vi "Configure Measurement Cursors.vi"(11 "State in":T2={"Graph Visible Items"={"Plot Legend"=FALSE, "Scale Legend"=FALSE, "Graph Palette"=FALSE, "Cursor Legend"=FALSE, "X Scrollbar"=FALSE}, "View Table"=FALSE, "Table Visible Items"={"Vertical Scrollbar"=FALSE, "Horizontal Scrollbar"=FALSE, "Row Headers"=FALSE, "Column Headers"=FALSE, "Vertical Lines"=FALSE, "Horizontal Lines"=FALSE}, "Header Font"={"Font Name"="", "Size"=0, "Bold"=FALSE, "Italic"=FALSE, "Underline"=FALSE, "Strikeout"=FALSE, "Color"=0}, "Cell Font"={"Font Name"="", "Size"=0, "Bold"=FALSE, "Italic"=FALSE, "Underline"=FALSE, "Strikeout"=FALSE, "Color"=0}, "Description and Tip..."={"Description"="", "Tip"=""}, "Moveable Splitter Position"=0, "Measurement Cursor Configuration"={"XY"={"enable XY"=FALSE, "Position (X)"=[], "Type"=enum."Absolute", "Y reference"=0.0, "color"=0}, "band"={"enable band"=FALSE, "B1"=0.0, "B2"=0.0, "Fixed bandwidth (B2-B1)"=0.0, "B1 color"=0, "B2 color"=0}, "harmonic"={"enable harmonics"=FALSE, "X reference (1X)"=0.0, "Maximum"=0, "Subset"=enum."All", "1X color"=0, "MX color"=0}, "sideband"={"enable sideband"=FALSE, "X center (C)"=0.0, "Sidebands"=0, "X spacing (s)"=0.0, "Center color"=0, "Sideband color"=0}}, "Cursors"={"List"=[], "Tags"=[]}, "X Increment"=0.0, "X Scale"={"Label Visible"=FALSE, "Label Text"="", "Mapping Mode"=0, "Format String"=""}, "Y Scale"={"Label Visible"=FALSE, "Label Text"="", "Mapping Mode"=0, "Format String"=""}, "Colors"={"background"=16777215, "major grid"=8355711, "minor grid"=12632256, "font"=0}, "desired spectrum view"={"scaling"={"linear/dB"=enum."no change", "dB reference"=0.0, "power/magnitude"=enum."no change", "view"=enum."no change"}, "spectral density"=enum."no change"}, "Plot Color Wheel"=[3381759, 32768, 982784, 4375295, 13827953, 13457919, 16757522, 4343295, 16728758, 12095254], "Plots"=[], "registered user events"=variant, "Lock 1X to Peak"=FALSE} caption="State" {"Y Scale"."Mapping Mode" items=["Linear", "Logarithmic", "dB"]; "X Scale"."Mapping Mode" items=["Linear", "Logarithmic"]}) -> (1 "OK":bool, 3 "State out":T2={"Graph Visible Items"={"Plot Legend"=FALSE, "Scale Legend"=FALSE, "Graph Palette"=FALSE, "Cursor Legend"=FALSE, "X Scrollbar"=FALSE}, "View Table"=FALSE, "Table Visible Items"={"Vertical Scrollbar"=FALSE, "Horizontal Scrollbar"=FALSE, "Row Headers"=FALSE, "Column Headers"=FALSE, "Vertical Lines"=FALSE, "Horizontal Lines"=FALSE}, "Header Font"={"Font Name"="", "Size"=0, "Bold"=FALSE, "Italic"=FALSE, "Underline"=FALSE, "Strikeout"=FALSE, "Color"=0}, "Cell Font"={"Font Name"="", "Size"=0, "Bold"=FALSE, "Italic"=FALSE, "Underline"=FALSE, "Strikeout"=FALSE, "Color"=0}, "Description and Tip..."={"Description"="", "Tip"=""}, "Moveable Splitter Position"=0, "Measurement Cursor Configuration"={"XY"={"enable XY"=FALSE, "Position (X)"=[], "Type"=enum."Absolute", "Y reference"=0.0, "color"=0}, "band"={"enable band"=FALSE, "B1"=0.0, "B2"=0.0, "Fixed bandwidth (B2-B1)"=0.0, "B1 color"=0, "B2 color"=0}, "harmonic"={"enable harmonics"=FALSE, "X reference (1X)"=0.0, "Maximum"=0, "Subset"=enum."All", "1X color"=0, "MX color"=0}, "sideband"={"enable sideband"=FALSE, "X center (C)"=0.0, "Sidebands"=0, "X spacing (s)"=0.0, "Center color"=0, "Sideband color"=0}}, "Cursors"={"List"=[], "Tags"=[]}, "X Increment"=0.0, "X Scale"={"Label Visible"=FALSE, "Label Text"="", "Mapping Mode"=0, "Format String"=""}, "Y Scale"={"Label Visible"=FALSE, "Label Text"="", "Mapping Mode"=0, "Format String"=""}, "Colors"={"background"=16777215, "major grid"=8355711, "minor grid"=12632256, "font"=0}, "desired spectrum view"={"scaling"={"linear/dB"=enum."no change", "dB reference"=0.0, "power/magnitude"=enum."no change", "view"=enum."no change"}, "spectral density"=enum."no change"}, "Plot Color Wheel"=[3381759, 32768, 982784, 4375295, 13827953, 13457919, 16757522, 4343295, 16728758, 12095254], "Plots"=[], "registered user events"=variant, "Lock 1X to Peak"=FALSE} caption="State" {"Y Scale"."Mapping Mode" items=["Linear", "Logarithmic", "dB"]; "X Scale"."Mapping Mode" items=["Linear", "Logarithmic"]})   [LabVIEW 2017, in "Octave with Cursors.xctl"]
doc: "Dialog for cursor configuration."
uses:
  <vilib>/addons/_XControls/Octave with Cursors/Octave with Cursors.xctl
  <vilib>/addons/_XControls/Octave with Cursors/Controls/State.ctl
  <vilib>/Utility/miscctls.llb/LVFontTypeDef.ctl
  <vilib>/addons/_XControls/Octave with Cursors/Controls/Measurement Cursor Configuration.ctl
panel:
  in  "XY color":u32(colorbox)
  in  "enable XY":bool
  in  "Type":enum16{"Absolute", "Relative"}(ring)
  in  "Position (i)":dbl[](array[numeric]) min=0.0 step=1.0
  in  "Y reference":dbl
  in  "B2 color":u32(colorbox)
  in  "B1 color":u32(colorbox)
  in  "Fixed ratio (octaves)":T1(ring)
  in  "enable band":bool
  in  "Stop (b2)":dbl=480.0
  in  "Start (b1)":dbl=20.0
  in  "1X color":u32(colorbox)
  in  "MX color":u32(colorbox)
  in  "enable harmonics":bool
  in  "Maximum (mX)":i32=10 min=2 max=99 step=1
  in  "X reference (1X)":dbl=60.0 min=0.001 step=1.0
  in  "Subset":enum16{"All", "Even", "Odd"}(ring)
  in  "Center color":u32(colorbox)
  in  "Sideband color":u32(colorbox)
  in  "Sidebands (sn)":i32=2 min=1 max=9 step=1
  in  "enable sideband":bool
  in  "X spacing (s)":dbl=60.0 min=0.0 step=1.0
  in  "X center (C)":dbl=8000.0 min=0.001 step=0.001
  in  "Cancel":bool
  in  "OK":bool
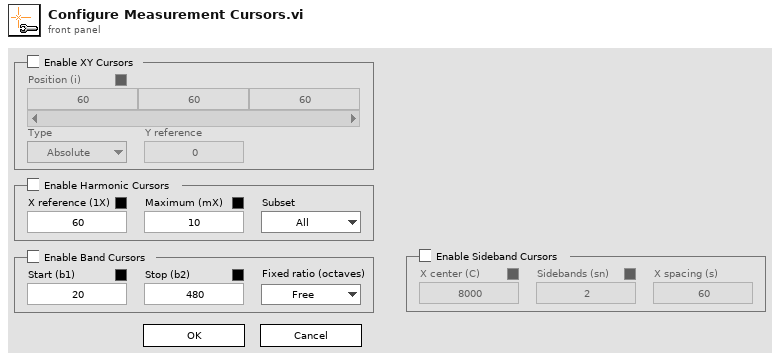
[diagram p1: front panel]
types:
  T1 = enum16{"Free", "1/24", "1/12", "1/6", "1/3", "1", "2", "4", "6", "8", "10"}
  T2 = typedef "Octave with Cursors.xctl/State.ctl" = cluster{"Graph Visible Items":cluster{"Plot Legend":bool, "Scale Legend":bool, "Graph Palette":bool, "Cursor Legend":bool, "X Scrollbar":bool}, "View Table":bool, "Table Visible Items":cluster{"Vertical Scrollbar":bool, "Horizontal Scrollbar":bool, "Row Headers":bool, "Column Headers":bool, "Vertical Lines":bool, "Horizontal Lines":bool}, "Header Font":T3, "Cell Font":T3, "Description and Tip...":cluster{"Description":string, "Tip":string}, "Moveable Splitter Position":i32, "Measurement Cursor Configuration":T4, "Cursors":cluster{"List":cluster{"Name":string, "Color":u32, "Style":i32, "Point Style":u8, "Name Visible":bool, "Allow Drag":bool, "Cursor Mode":u32, "Plot":i32, "Index":i32, "Position":cluster{"X":dbl, "Y":dbl}, "X Scale":u32, "Y Scale":u32, "Watch Plots":i32[], "Watch All Plots":bool, "Plot Area":i32, "Label Offset":cluster{"X":dbl, "Y":dbl}}[], "Tags":variant[]}, "X Increment":dbl, "X Scale":cluster{"Label Visible":bool, "Label Text":string, "Mapping Mode":u8, "Format String":string}, "Y Scale":cluster{"Label Visible":bool, "Label Text":string, "Mapping Mode":u8, "Format String":string}, "Colors":cluster{"background":u32, "major grid":u32, "minor grid":u32, "font":u32}, "desired spectrum view":cluster{"scaling":cluster{"linear/dB":enum16{"no change", "linear", "dB"}, "dB reference":dbl, "power/magnitude":enum16{"no change", "power", "magnitude"}, "view":enum16{"no change", "rms", "peak", "peak-peak"}}, "spectral density":enum16{"no change", "spectrum", "spectral density"}}, "Plot Color Wheel":u32[], "Plots":cluster{"Name":string, "Line Color":u32, "Line Style":u8, "Line Width":u8, "Fill/Point Color":u32, "Point Style":u8, "Fill To":i16, "Interpolation":u8, "Anti-aliased":bool}[], "registered user events":variant, "Lock 1X to Peak":bool}
  T3 = typedef "LVFontTypeDef.ctl" = cluster{"Font Name":string, "Size":u16, "Bold":bool, "Italic":bool, "Underline":bool, "Strikeout":bool, "Color":u32}
  T4 = typedef "Octave with Cursors.xctl/Measurement Cursor Configuration.ctl" = cluster{"XY":cluster{"enable XY":bool, "Position (X)":dbl[], "Type":enum16{"Absolute", "Relative"}, "Y reference":dbl, "color":u32}, "band":cluster{"enable band":bool, "B1":dbl, "B2":dbl, "Fixed bandwidth (B2-B1)":dbl, "B1 color":u32, "B2 color":u32}, "harmonic":cluster{"enable harmonics":bool, "X reference (1X)":dbl, "Maximum":i32, "Subset":enum16{"All", "Even", "Odd"}, "1X color":u32, "MX color":u32}, "sideband":cluster{"enable sideband":bool, "X center (C)":dbl, "Sidebands":i32, "X spacing (s)":dbl, "Center color":u32, "Sideband color":u32}}
  T5 = cluster{"enable XY":bool, "Position (X)":dbl[], "Type":enum16{"Absolute", "Relative"}, "Y reference":dbl, "color":u32}
  T6 = cluster{"enable harmonics":bool, "X reference (1X)":dbl, "Maximum":i32, "Subset":enum16{"All", "Even", "Odd"}, "1X color":u32, "MX color":u32}
  T7 = cluster{"enable sideband":bool, "X center (C)":dbl, "Sidebands":i32, "X spacing (s)":dbl, "Center color":u32, "Sideband color":u32}
  T8 = cluster{"enable band":bool, "B1":dbl, "B2":dbl, "Fixed bandwidth (B2-B1)":dbl, "B1 color":u32, "B2 color":u32}
  T9 = enum8{"Enabled", "Disabled", "Disabled and Grayed Out"}
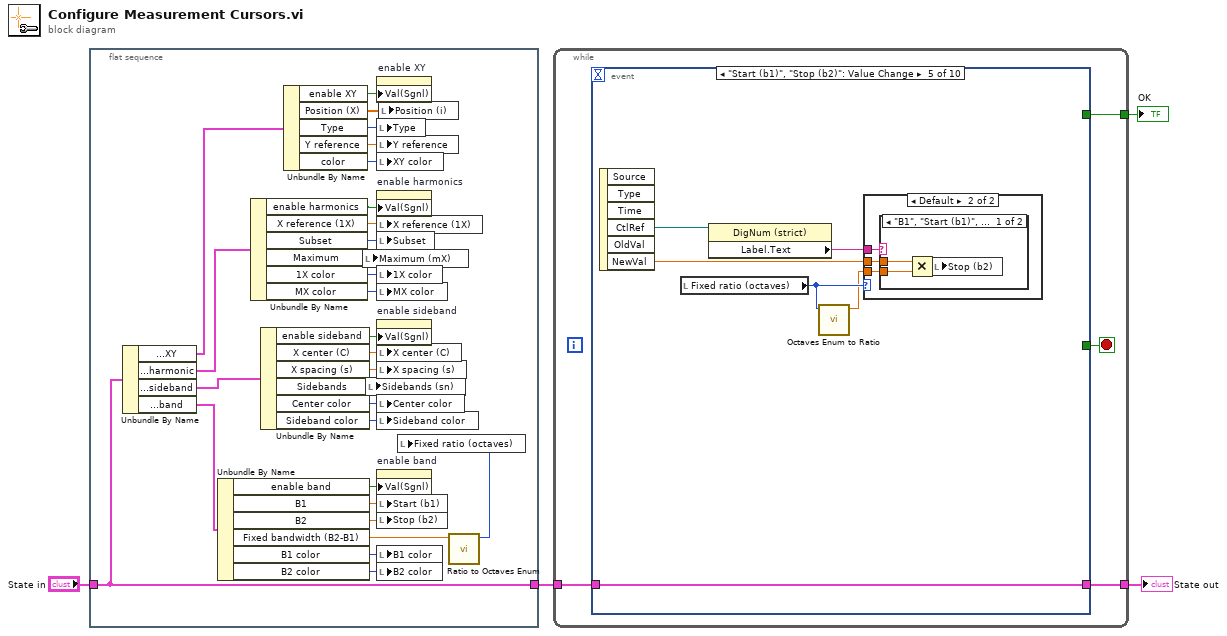
[diagram p0: block diagram]
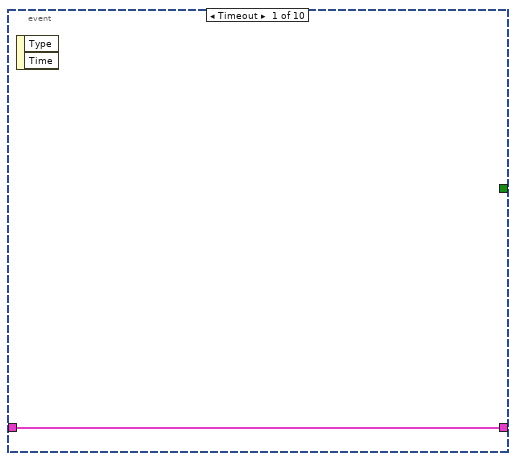
[diagram p2: hidden frame]
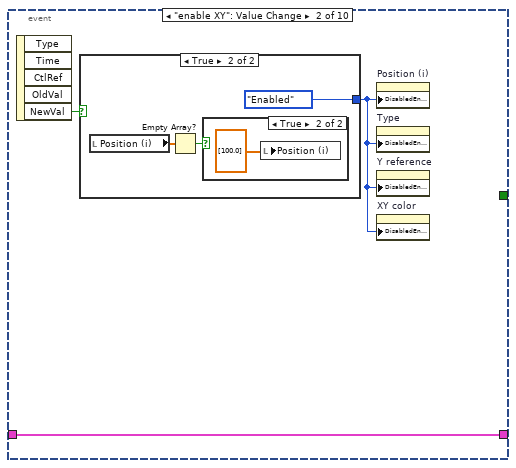
[diagram p3: hidden frame]
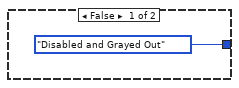
[diagram p4: hidden frame]
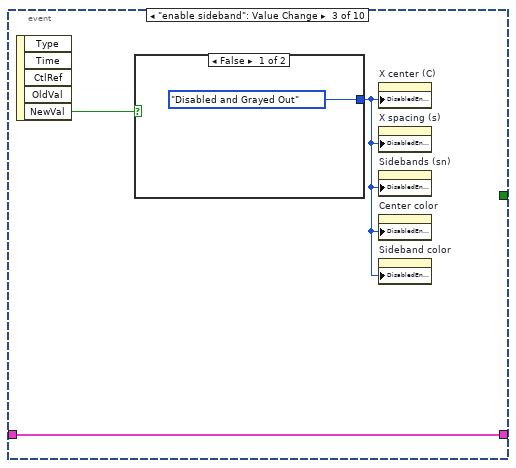
[diagram p6: hidden frame]
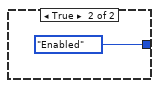
[diagram p7: hidden frame]
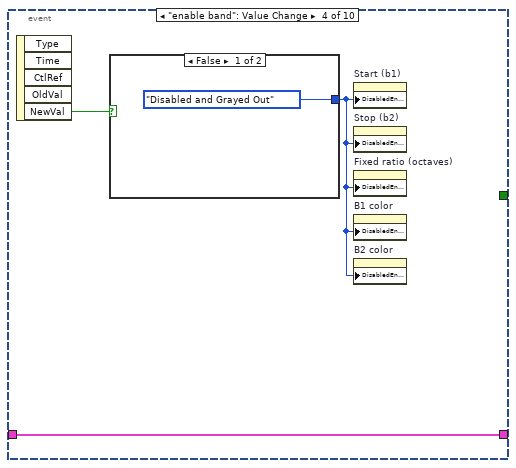
[diagram p8: hidden frame]
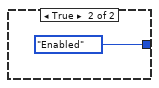
[diagram p9: hidden frame]
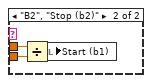
[diagram p11: hidden frame]
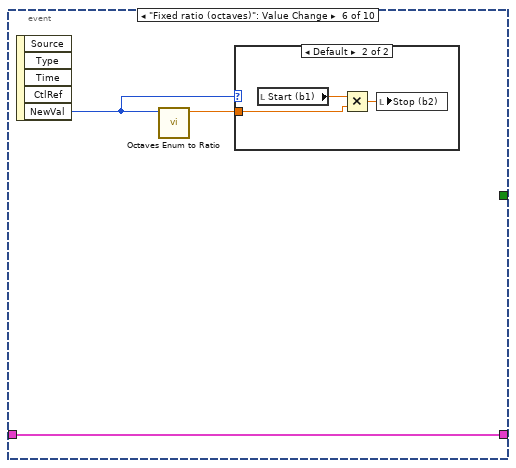
[diagram p12: hidden frame]
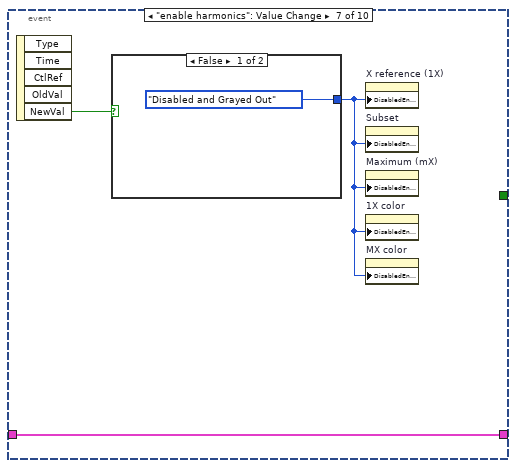
[diagram p14: hidden frame]
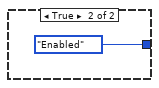
[diagram p15: hidden frame]
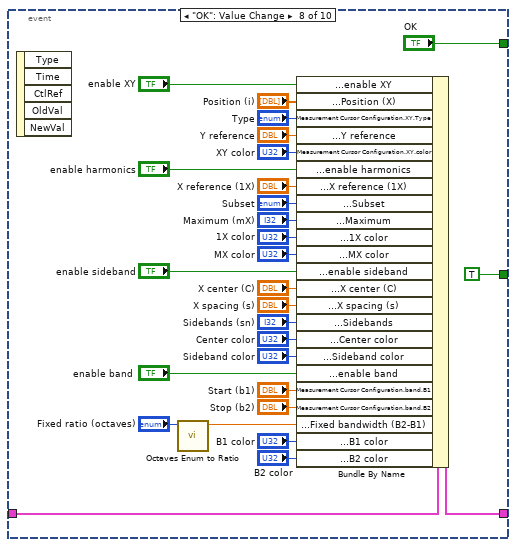
[diagram p16: hidden frame]
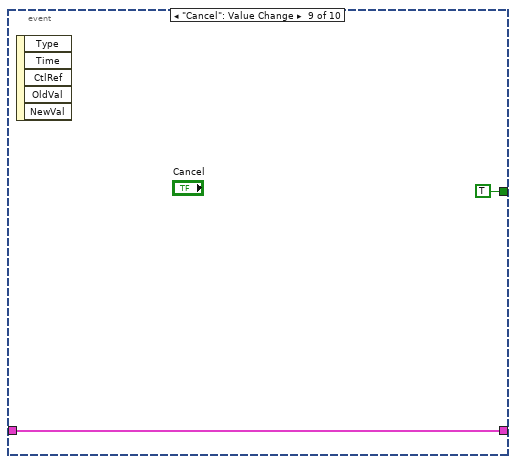
[diagram p17: hidden frame]
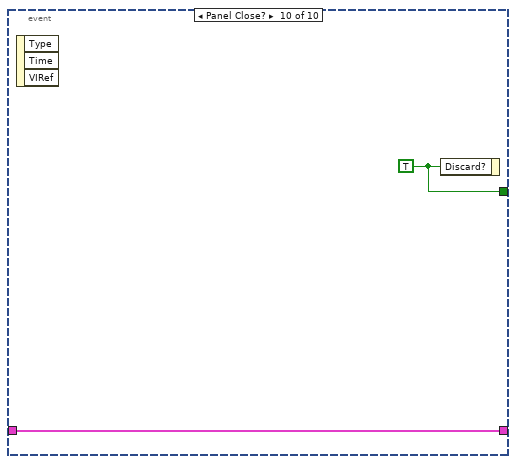
[diagram p18: hidden frame]
diagram:
  n1 = flat-sequence {
    tunnel: "State in" -> [w18]
    tunnel: [w18] -> w2
    frame #0 {
      n2 = Unbundle By Name(w18) -> ("Measurement Cursor Configuration.XY"=w33:T5, "Measurement Cursor Configuration.harmonic"=w29:T6, "Measurement Cursor Configuration.sideband"=w25:T7, "Measurement Cursor Configuration.band"=w21:T8)
      n3 = Unbundle By Name(w21) -> ("enable band"=w14:bool, "B1"=w20:dbl, "B2"=w19:dbl, "Fixed bandwidth (B2-B1)"=w6:dbl, "B1 color"=w8:u32, "B2 color"=w7:u32)
      n4 = Unbundle By Name(w29) -> ("enable harmonics"=w16:bool, "X reference (1X)"=w28:dbl, "Subset"=w27:enum16{"All", "Even", "Odd"}, "Maximum"=w26:i32, "1X color"=w12:u32, "MX color"=w11:u32)
      n5 = Unbundle By Name(w25) -> ("enable sideband"=w15:bool, "X center (C)"=w24:dbl, "X spacing (s)"=w23:dbl, "Sidebands"=w22:i32, "Center color"=w10:u32, "Sideband color"=w9:u32)
      n6 = Unbundle By Name(w33) -> ("enable XY"=w17:bool, "Position (X)"=w32:dbl[], "Type"=w31:enum16{"Absolute", "Relative"}, "Y reference"=w30:dbl, "color"=w13:u32)
      n7 = local write "Maximum (mX)"(w26) -> ()
      n8 = local write "Sidebands (sn)"(w22) -> ()
      n9 = property on="enable XY" class="Bool (strict)"("Val(Sgnl)"=w17) -> ()  [unwired: 2 in, 2 out]
      n10 = local write "Type"(w31) -> ()
      n11 = local write "Y reference"(w30) -> ()
      n12 = local write "XY color"(w13) -> ()
      n13 = property on="enable harmonics" class="Bool (strict)"("Val(Sgnl)"=w16) -> ()  [unwired: 2 in, 2 out]
      n14 = local write "X reference (1X)"(w28) -> ()
      n15 = local write "Subset"(w27) -> ()
      n16 = local write "1X color"(w12) -> ()
      n17 = local write "MX color"(w11) -> ()
      n18 = property on="enable sideband" class="Bool (strict)"("Val(Sgnl)"=w15) -> ()  [unwired: 2 in, 2 out]
      n19 = local write "X center (C)"(w24) -> ()
      n20 = local write "X spacing (s)"(w23) -> ()
      n21 = local write "Center color"(w10) -> ()
      n22 = local write "Sideband color"(w9) -> ()
      n23 = property on="enable band" class="Bool (strict)"("Val(Sgnl)"=w14) -> ()  [unwired: 2 in, 2 out]
      n24 = local write "Start (b1)"(w20) -> ()
      n25 = local write "Stop (b2)"(w19) -> ()
      n26 = local write "B1 color"(w8) -> ()
      n27 = local write "B2 color"(w7) -> ()
      n28 = local write "Position (i)"(w32) -> ()
      n29 = call <vilib>:"Ratio to Octaves Enum.vi"("ratio"=w6) -> ("octaves"=w5:T1)  [unwired: 10 in]
      n30 = local write "Fixed ratio (octaves)"(w5) -> ()
    }
  }
  n31 = while {
    tunnel: w2 -> [w35]
    tunnel: [w36] -> w4
    tunnel: [w34] -> w1
    stop <- w37 stop-if-true
    n32 = event shown="[4] \"Start (b1)\", \"Stop (b2)\": Value Change" {
      selector: _ -> [_ _ _ _ _ _ _ _ _ _]
      dyn-events: _ -> [_ _ _ _ _ _ _ _ _ _]
      timeout: _ -> [_ _ _ _ _ _ _ _ _ _]
      tunnel: [_ _ _ _ _ _ _ TRUE TRUE w113] -> w37
      tunnel: [w38 w40 w48 w53 w62 w74 w79 w96 w111 w114] -> w36
      tunnel: w35 -> [w38 w40 w48 w53 w62 w74 w79 w97 w111 w114]
      tunnel: [_ _ _ _ _ _ _ "OK" _ _] -> w34
      event Timeout {
        n33 = event-data() -> ()  [unwired: 1 in, 2 out]
      }
      event "enable XY": Value Change {
        n34 = event-data() -> ("NewVal"=w41:bool)  [unwired: 1 in, 4 out]
        n35 = case shown="True" w41 {
          tunnel: [T9."Disabled and Grayed Out" ("Disabled") T9."Enabled" ("Disabled")] -> w39
          frame False {
          }
          frame True {
            n36 = local read "Position (i)"() -> (w44:dbl[])
            n37 = Empty Array?(array=w44) -> (empty?=w43:bool)
            n38 = case shown="True" w43 {
              frame False {
              }
              frame True {
                n39 = local write "Position (i)"(dbl[] [100.0] ("Position (i)")) -> ()
              }
            }
          }
        }
        n40 = property on="Position (i)" class="Arr (strict)"("DisabledEnum"=w39) -> ()  [unwired: 2 in, 2 out]
        n41 = property on="Type" class="Enum (strict)"("DisabledEnum"=w39) -> ()  [unwired: 2 in, 2 out]
        n42 = property on="Y reference" class="DigNum (strict)"("DisabledEnum"=w39) -> ()  [unwired: 2 in, 2 out]
        n43 = property on="XY color" class="ColBox"("DisabledEnum"=w39) -> ()  [unwired: 2 in, 2 out]
      }
      event "enable sideband": Value Change {
        n44 = event-data() -> ("NewVal"=w49:bool)  [unwired: 1 in, 4 out]
        n45 = case shown="False" w49 {
          tunnel: [T9."Disabled and Grayed Out" ("Disabled") T9."Enabled" ("Disabled")] -> w47
          frame False {
          }
          frame True {
          }
        }
        n46 = property on="X center (C)" class="DigNum (strict)"("DisabledEnum"=w47) -> ()  [unwired: 2 in, 2 out]
        n47 = property on="X spacing (s)" class="DigNum (strict)"("DisabledEnum"=w47) -> ()  [unwired: 2 in, 2 out]
        n48 = property on="Sidebands (sn)" class="DigNum (strict)"("DisabledEnum"=w47) -> ()  [unwired: 2 in, 2 out]
        n49 = property on="Center color" class="ColBox"("DisabledEnum"=w47) -> ()  [unwired: 2 in, 2 out]
        n50 = property on="Sideband color" class="ColBox"("DisabledEnum"=w47) -> ()  [unwired: 2 in, 2 out]
      }
      event "enable band": Value Change {
        n51 = event-data() -> ("NewVal"=w54:bool)  [unwired: 1 in, 4 out]
        n52 = case shown="False" w54 {
          tunnel: [T9."Disabled and Grayed Out" ("Disabled") T9."Enabled" ("Disabled")] -> w52
          frame False {
          }
          frame True {
          }
        }
        n53 = property on="Start (b1)" class="DigNum (strict)"("DisabledEnum"=w52) -> ()  [unwired: 2 in, 2 out]
        n54 = property on="Stop (b2)" class="DigNum (strict)"("DisabledEnum"=w52) -> ()  [unwired: 2 in, 2 out]
        n55 = property on="Fixed ratio (octaves)" class="Enum (strict)"("DisabledEnum"=w52) -> ()  [unwired: 2 in, 2 out]
        n56 = property on="B1 color" class="ColBox"("DisabledEnum"=w52) -> ()  [unwired: 2 in, 2 out]
        n57 = property on="B2 color" class="ColBox"("DisabledEnum"=w52) -> ()  [unwired: 2 in, 2 out]
      }
      event "Start (b1)", "Stop (b2)": Value Change {
        n58 = event-data() -> ("CtlRef"=w60:refnum<vi>, "NewVal"=w59:dbl)  [unwired: 1 in, 4 out]
        n59 = local read "Fixed ratio (octaves)"() -> (w58:T1)
        n60 = property class="DigNum (strict)"(reference=w60) -> ("Label.Text"=w61:string)  [unwired: 1 in, 2 out]
        n61 = call <vilib>:"Octaves Enum to Ratio.vi"("octaves"=w58) -> ("ratio"=w57:dbl)  [unwired: 10 in]
        n62 = case shown="Default" w58 {
          tunnel: w61 -> [_ w65]
          tunnel: w59 -> [_ w64]
          tunnel: w57 -> [_ w63]
          frame "Free" {
          }
          frame Default {
            n63 = case shown="\"B1\", \"Start (b1)\", Default" w65 {
              tunnel: w64 -> [w68 w71]
              tunnel: w63 -> [w67 w70]
              frame "B1", "Start (b1)", Default {
                n64 = Multiply(x=w68, y=w67) -> (x*y=w66:dbl)
                n65 = local write "Stop (b2)"(w66) -> ()
              }
              frame "B2", "Stop (b2)" {
                n66 = Divide(x=w71, y=w70) -> (x/y=w69:dbl)
                n67 = local write "Start (b1)"(w69) -> ()
              }
            }
          }
        }
      }
      event "Fixed ratio (octaves)": Value Change {
        n68 = event-data() -> ("NewVal"=w72:T1)  [unwired: 1 in, 4 out]
        n69 = call <vilib>:"Octaves Enum to Ratio.vi"("octaves"=w72) -> ("ratio"=w73:dbl)  [unwired: 10 in]
        n70 = case shown="Default" w72 {
          tunnel: w73 -> [_ w77]
          frame "Free" {
          }
          frame Default {
            n71 = local read "Start (b1)"() -> (w76:dbl)
            n72 = Multiply(x=w76, y=w77) -> (x*y=w75:dbl)
            n73 = local write "Stop (b2)"(w75) -> ()
          }
        }
      }
      event "enable harmonics": Value Change {
        n74 = event-data() -> ("NewVal"=w80:bool)  [unwired: 1 in, 4 out]
        n75 = case shown="False" w80 {
          tunnel: [T9."Disabled and Grayed Out" ("Disabled") T9."Enabled" ("Disabled")] -> w78
          frame False {
          }
          frame True {
          }
        }
        n76 = property on="X reference (1X)" class="DigNum (strict)"("DisabledEnum"=w78) -> ()  [unwired: 2 in, 2 out]
        n77 = property on="Subset" class="Enum (strict)"("DisabledEnum"=w78) -> ()  [unwired: 2 in, 2 out]
        n78 = property on="Maximum (mX)" class="DigNum (strict)"("DisabledEnum"=w78) -> ()  [unwired: 2 in, 2 out]
        n79 = property on="1X color" class="ColBox"("DisabledEnum"=w78) -> ()  [unwired: 2 in, 2 out]
        n80 = property on="MX color" class="ColBox"("DisabledEnum"=w78) -> ()  [unwired: 2 in, 2 out]
      }
      event "OK": Value Change {
        n81 = event-data() -> ()  [unwired: 1 in, 5 out]
        n82 = call <vilib>:"Octaves Enum to Ratio.vi"("octaves"="Fixed ratio (octaves)") -> ("ratio"=w83:dbl)  [unwired: 10 in]
        n83 = Bundle By Name(cluster=w97, "Measurement Cursor Configuration.XY.enable XY"="enable XY", "Measurement Cursor Configuration.XY.Position (X)"="Position (i)", "Measurement Cursor Configuration.XY.Type"="Type", "Measurement Cursor Configuration.XY.Y reference"="Y reference", "Measurement Cursor Configuration.XY.color"="XY color", "Measurement Cursor Configuration.harmonic.enable harmonics"="enable harmonics", "Measurement Cursor Configuration.harmonic.X reference (1X)"="X reference (1X)", "Measurement Cursor Configuration.harmonic.Subset"="Subset", "Measurement Cursor Configuration.harmonic.Maximum"="Maximum (mX)", "Measurement Cursor Configuration.harmonic.1X color"="1X color", "Measurement Cursor Configuration.harmonic.MX color"="MX color", "Measurement Cursor Configuration.sideband.enable sideband"="enable sideband", "Measurement Cursor Configuration.sideband.X center (C)"="X center (C)", "Measurement Cursor Configuration.sideband.X spacing (s)"="X spacing (s)", "Measurement Cursor Configuration.sideband.Sidebands"="Sidebands (sn)", "Measurement Cursor Configuration.sideband.Center color"="Center color", "Measurement Cursor Configuration.sideband.Sideband color"="Sideband color", "Measurement Cursor Configuration.band.enable band"="enable band", "Measurement Cursor Configuration.band.B1"="Start (b1)", "Measurement Cursor Configuration.band.B2"="Stop (b2)", "Measurement Cursor Configuration.band.Fixed bandwidth (B2-B1)"=w83, "Measurement Cursor Configuration.band.B1 color"="B1 color", "Measurement Cursor Configuration.band.B2 color"="B2 color") -> (w96:T2)
      }
      event "Cancel": Value Change {
        n84 = event-data() -> ()  [unwired: 1 in, 5 out]
      }
      event Panel Close? {
        w113 = TRUE
        n85 = event-data() -> ()  [unwired: 1 in, 3 out]
        n86 = event-data("Discard?"=w113) -> ()  [unwired: 1 in, 1 out]
      }
    }
  }
  "State out" <- w4
  "OK" <- w1
